vi "20220107_HW00_WaveGenerator.vi"(1 "Time":i32, 2 "Wave Size":i32=15, 3 "Coords":cluster{"Numeric":i32, "Numeric":i32}={"Numeric"=50, "Numeric"=50}, 4 "Graph Size":i32=100) -> (0 "Graph":dbl[][](graph))   [LabVIEW 2019]
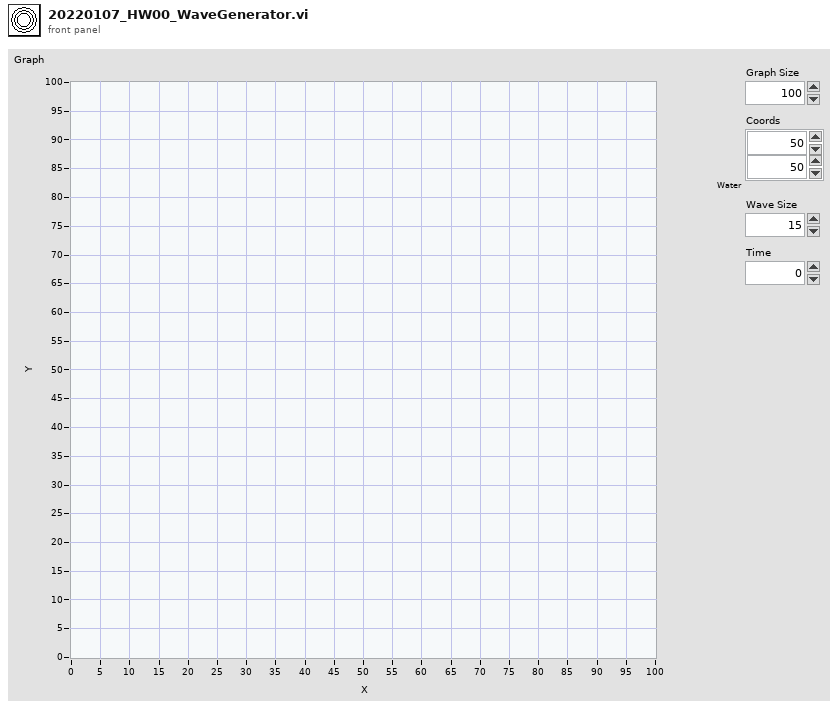
[diagram p1: front panel]
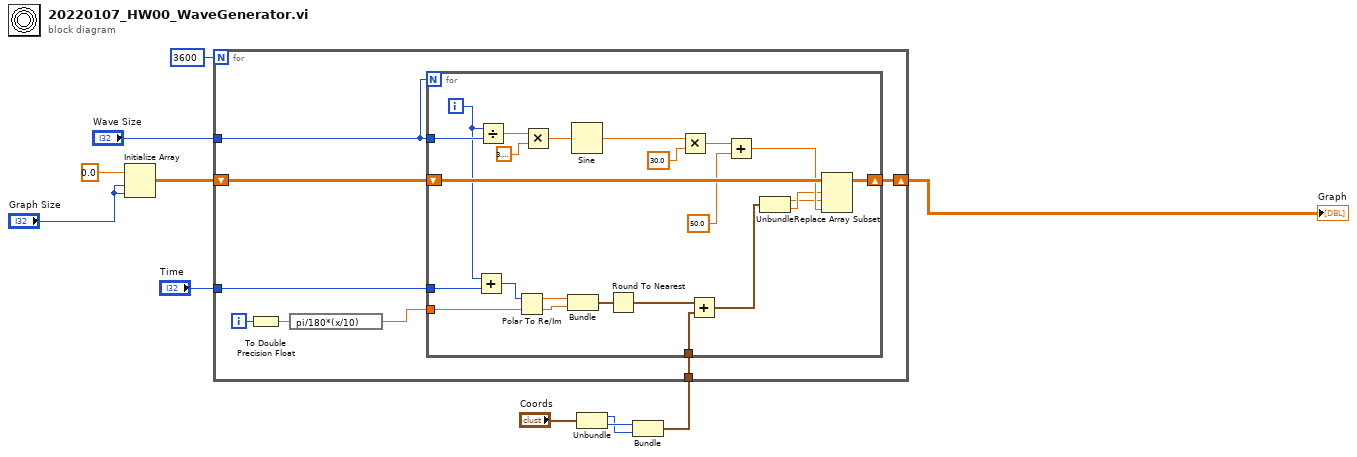
[diagram p0: block diagram]
diagram:
  n1 = Initialize Array(0.0, "Graph Size", "Graph Size") -> (w9:dbl[][])
  n2 = Unbundle("Coords") -> ("Numeric"=w2:i32, "Numeric"=w3:i32)
  n3 = Bundle("Numeric"=w3, "Numeric"=w2) -> (w1:cluster{"Numeric":i32, "Numeric":i32})  [unwired: 1 in]
  n4 = for {
    N: 3600 -> [_]
    shift-right: [w18] -> w8
    shift-left: w9 -> [w19]
    tunnel: w1 -> [w14]
    tunnel: "Time" -> [w13]
    tunnel: "Wave Size" -> [w12]
    i -> [w17]
    n5 = To Double Precision Float(number=w17) -> (double precision float=w16:dbl)
    n6 = expression code="pi/180*(x/10)"(w16) -> (w15:dbl)
    n7 = for {
      N: w12 -> [_]
      shift-right: [w41] -> w18
      shift-left: w19 -> [w42]
      tunnel: w12 -> [w32]
      tunnel: w15 -> [w31]
      tunnel: w14 -> [w28]
      tunnel: w13 -> [w22]
      i -> [w24]
      n8 = Add(x=w24, y=w22) -> (x+y=w23:i32)
      n9 = Divide(x=w24, y=w32) -> (x/y=w40:dbl)
      n10 = Polar To Re/Im(2:w31, 3:w23) -> (0:w29:dbl, 1:w30:dbl)
      n11 = Multiply(x=w40, y=3.141592653589793) -> (x*y=w35:dbl)
      n12 = Bundle(w30, w29) -> (w21:cluster{dbl, dbl})  [unwired: 1 in]
      n13 = Sine(x=w35) -> (sin(x)=w34:dbl)
      n14 = Round To Nearest(number=w21) -> (nearest integer value=w20:cluster{dbl, dbl})
      n15 = Multiply(x=w34, y=30.0 ("new element/subarray")) -> (x*y=w37:dbl)
      n16 = Add(x=w20, y=w28) -> (x+y=w27:cluster{dbl, dbl})
      n17 = Add(x=w37, y=50.0 ("new element/subarray")) -> (x+y=w33:dbl)
      n18 = Unbundle(w27) -> (w25:dbl, w26:dbl)
      n19 = Replace Array Subset(array=w42, new element=w33, index (row)=w26, index (col)=w25) -> (w41:dbl[][])
    }
  }
  "Graph" <- w8
